vi "Write State.vi"(8 "error in (no error)":errorcluster, 10 "State":refnum<class "State Pattern.lvclass">, 11 "Context Actor in":refnum<class "Context Actor.lvclass">) -> (0 "error out":errorcluster, 3 "Context Actor out":refnum<class "Context Actor.lvclass">)   [LabVIEW 2021, in "Context Actor.lvlib" / "Context Actor.lvclass"]
uses:
  Context Actor.lvclass
  Context Actor.lvclass/Context Actor.ctl
  Context State/Context State.lvclass
  State Pattern/State Pattern.lvclass
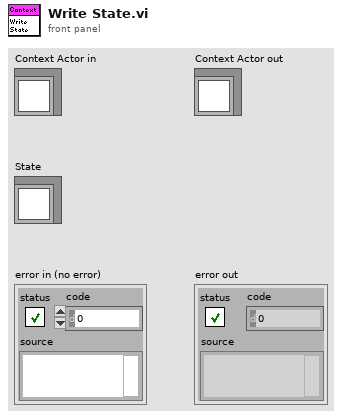
[diagram p1: front panel]
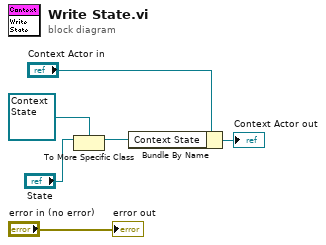
[diagram p0: block diagram]
diagram:
  n1 = To More Specific Class(target class=refnum<class "Context State.lvclass"> refnum ("Context Actor.lvlib:Context State.lvclass"), reference="State") -> (specific class reference=w2:refnum<class "Context State.lvclass">)  [unwired: 1 in, 1 out]
  n2 = Bundle By Name(cluster="Context Actor in", "Context State"=w2) -> (→"Context Actor out":refnum<class "Context Actor.lvclass">)
  "error out" <- "error in (no error)"
